vi "Do Zig Zag.vi"(6 "Go to point right":dbl=500.0, 7 "Go to point left":dbl, 9 "Wall Left?":bool, 10 "Threshold Right":dbl=350.0, 11 "Threshold Left":dbl=150.0) -> (1 "Numeric":dbl, 2 "Numeric 2":dbl, 3 "Wall error 2":dbl)   [LabVIEW 2017]
uses:
  Globals/Pose.vi
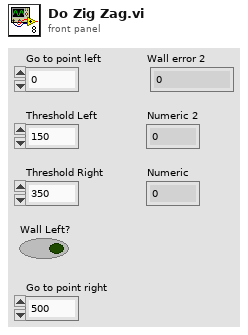
[diagram p1: front panel]
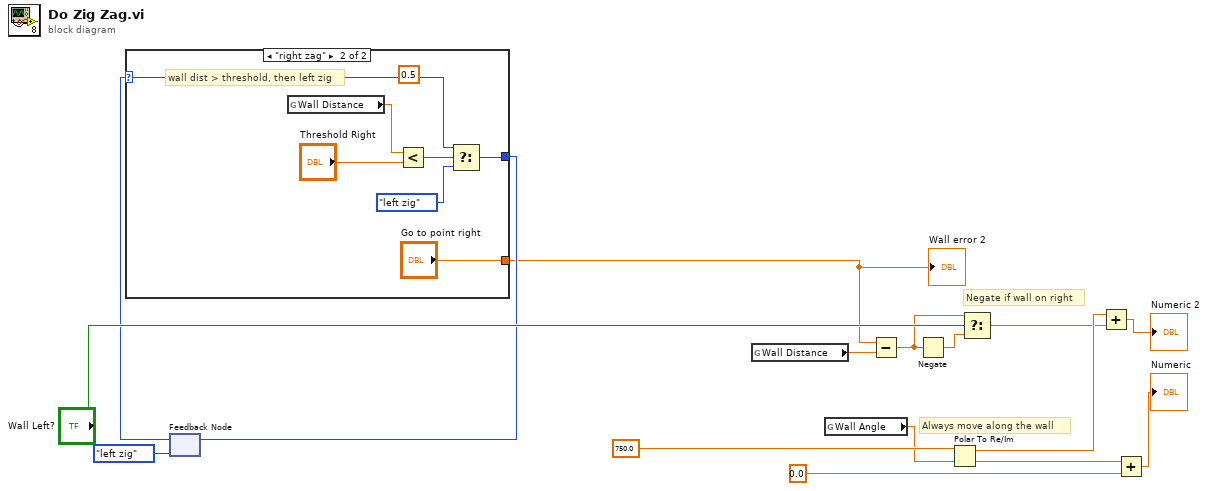
[diagram p0: block diagram]
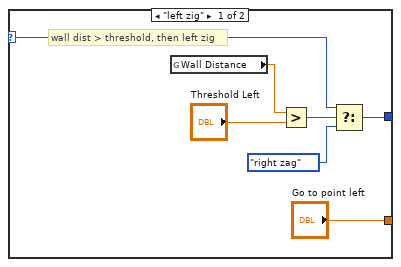
[diagram p2: hidden frame]
diagram:
  (unwired) 0.5
  # "Always move along the wall"
  # "Negate if wall on right"
  n1 = feedback #1(enum16{"left zig", "right zag"}."left zig" ("Zig or Zag")) -> (w4:enum16{"left zig", "right zag"})
  n2 = case shown="\"right zag\"" w4 {
    selector: w4 -> [w21 w26]
    tunnel: [w20 w27] -> w13
    tunnel: ["Go to point left" "Go to point right"] -> w2
    frame "left zig" {
      # "wall dist > threshold, then left zig"
      n3 = global read "Pose.vi" "Wall Distance"() -> (w22:dbl)
      n4 = Greater?(x=w22, y="Threshold Left") -> (0:w23:bool)
      n5 = Select(t=w21, s=w23, f=enum16{"left zig", "right zag"}."right zag" ("Zig or Zag")) -> (s? t:f=w20:enum16{"left zig", "right zag"})
    }
    frame "right zag" {
      # "wall dist > threshold, then left zig"
      n6 = global read "Pose.vi" "Wall Distance"() -> (w29:dbl)
      n7 = Less?(x=w29, y="Threshold Right") -> (x < y?=w30:bool)
      n8 = Select(t=w26, s=w30, f=enum16{"left zig", "right zag"}."left zig" ("Zig or Zag")) -> (s? t:f=w27:enum16{"left zig", "right zag"})
    }
  }
  "Wall error 2" <- w2
  n9 = feedback-in #1(w13) -> ()
  n10 = global read "Pose.vi" "Wall Distance"() -> (w3:dbl)
  n11 = global read "Pose.vi" "Wall Angle"() -> (w6:dbl)
  n12 = Subtract(x=w2, y=w3) -> (x-y=w1:dbl)
  n13 = Negate(x=w1) -> (-x=w9:dbl)
  n14 = Polar To Re/Im(2:w6, 3:750.0 ("r")) -> (0:w8:dbl, 1:w7:dbl)
  n15 = Select(t=w1, s="Wall Left?", f=w9) -> (s? t:f=w5:dbl)
  n16 = Add(x=w7, y=w5) -> (x+y=→"Numeric 2":dbl)
  n17 = Add(x=w8, y=0.0) -> (x+y=→"Numeric":dbl)
